vi "Clear.vi"(8 "error in (no error)":errorcluster, 11 "Debug View In":refnum<class "Debug View.lvclass">) -> (0 "error out":errorcluster)   [LabVIEW 2020, in "Debug View.lvclass"]
doc: "Clears any resorces allocated during initialization."
uses:
  Debug View.lvclass
  Debug View.lvclass/Debug View.ctl
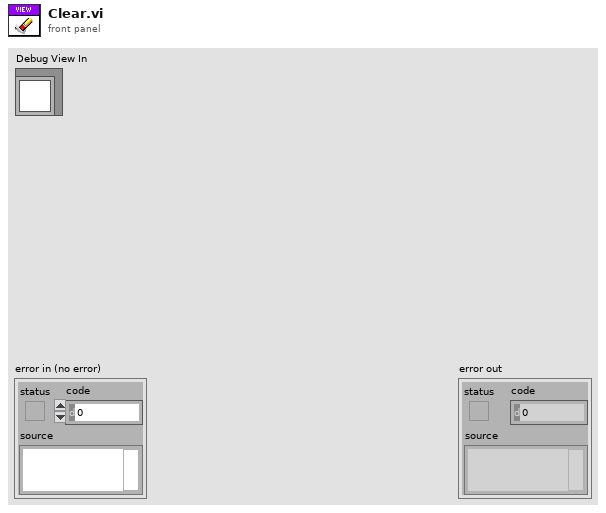
[diagram p1: front panel]
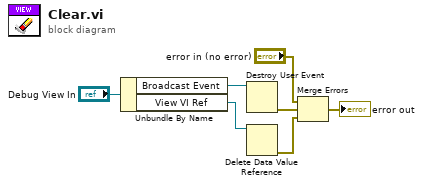
[diagram p0: block diagram]
diagram:
  n1 = Unbundle By Name("Debug View In") -> ("Broadcast Event"=w4:refnum<user-event>, "View VI Ref"=w2:refnum<data-value>)
  n2 = Destroy User Event(user event=w4) -> (error out=w3:errorcluster)  [unwired: 1 in]
  n3 = Delete Data Value Reference(data value reference=w2) -> (error out=w1:errorcluster)  [unwired: 1 in, 1 out]
  n4 = Merge Errors("error in (no error)", w3, w1) -> (→"error out":errorcluster)
